vi "Cryo-Con Set T.vi"(8 "error in (no error)":errorcluster, 9 "Output #":i32=1, 10 "Set T":dbl=2.0, 11 "VISA Resource Name":refnum<visa-resource-name>) -> (0 "error out":errorcluster, 3 "VISA Resource Name Out":refnum<visa-resource-name>)   [LabVIEW 2021]
panel:
  out "resulting string":string
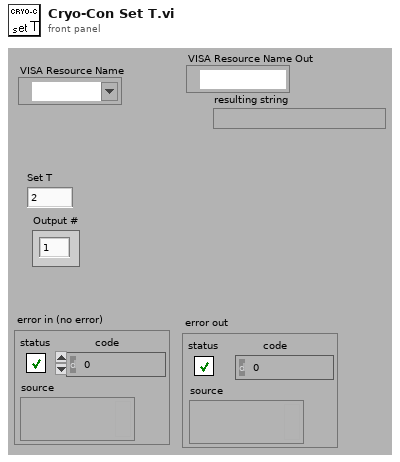
[diagram p1: front panel]
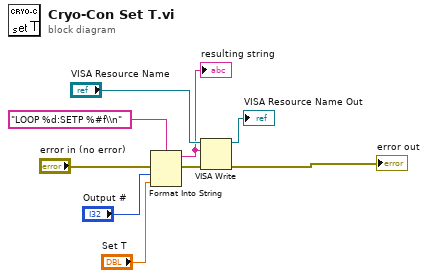
[diagram p0: block diagram]
diagram:
  n1 = Format Into String(format string="LOOP %d:SETP %#f\\n", error in="error in (no error)", "Output #", "Set T") -> (resulting string=w3:string, error out=w7:errorcluster)  [unwired: 1 in]
  "resulting string" <- w3
  n2 = VISA Write(VISA resource name="VISA Resource Name", write buffer=w3, error in (no error)=w7) -> (VISA resource name out=→"VISA Resource Name Out":refnum<visa-resource-name>, error out=→"error out":errorcluster)  [unwired: 1 out]
